vi "Find Invalid Group Settings.vi"(8 "error in (no error)":errorcluster, 11 "dsf refnum":T1) -> (0 "error out":errorcluster, 1 "Invalid Settings":string[](array[string]), 3 "dsf refnum out":T1)   [LabVIEW 2017, in "DSF Configuration.lvlib"]
uses:
  DSF Configuration.lvlib
  Controls/DSF Config Data RefNum.ctl
  Read All Item IDs/Read All Group IDs.vi
  Read Item Settings ID/Read Group Settings ID.vi
  Read All Item IDs/Read All Settings IDs.vi
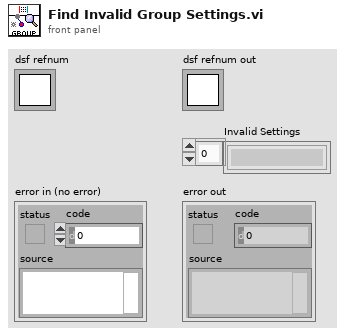
[diagram p1: front panel]
types:
  T1 = typedef "DSF Configuration.lvlib/DSF Config Data RefNum.ctl" = refnum<k1>
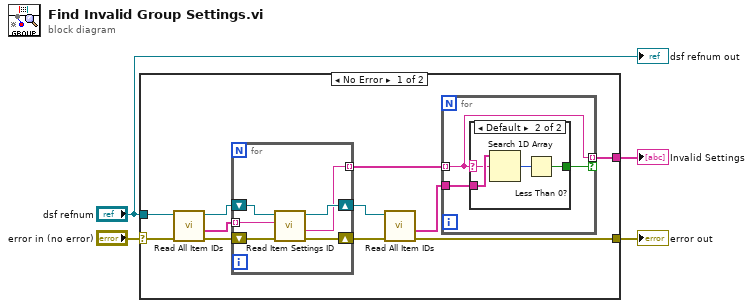
[diagram p0: block diagram]
diagram:
  n1 = case shown="No Error" "error in (no error)" {
    selector: "error in (no error)" -> [w15 w29]
    tunnel: "dsf refnum" -> [w14 _]
    tunnel: [w11 w29] -> w2
    tunnel: [w12 _] -> w1
    frame No Error {
      n2 = call-poly "Read All Item IDs.vi"("error in (no error)"=w15, "dsf refnum"=w14) -> ("error out"=w8:errorcluster, "Group IDs"=w6:string[], "dsf refnum out"=w10:T1)  [unwired: 7 in]
      n3 = for {
        shift-right: [w20] -> w9
        shift-left: w10 -> [w21]
        shift-right: [w18] -> w7
        shift-left: w8 -> [w19]
        tunnel: w6 -> [w17] mode=indexing
        tunnel: [w16] -> w5 mode=indexing
        n4 = call-poly "Read Item Settings ID.vi"("error in (no error)"=w19, "Group ID"=w17, "dsf refnum"=w21) -> ("error out"=w18:errorcluster, "Settings ID"=w16:string, "dsf refnum out"=w20:T1)  [unwired: 5 in, 1 out]
      }
      n5 = call-poly "Read All Item IDs.vi"("error in (no error)"=w7, "dsf refnum"=w9) -> ("error out"=w11:errorcluster, "Setting IDs"=w13:string[])  [unwired: 7 in, 1 out]
      n6 = for {
        tunnel: w5 -> [w23] mode=indexing
        tunnel: w13 -> [w24]
        tunnel: [w23] -> w12 mode=indexing if=w22
        n7 = case shown="Default" w23 {
          selector: w23 -> [_ w26]
          tunnel: w24 -> [_ w28]
          tunnel: [_ w25] -> w22
          frame "" {
          }
          frame Default {
            n8 = Search 1D Array(1D array=w28, element=w26) -> (index of element=w27:i32)  [unwired: 1 in]
            n9 = Less Than 0?(x=w27) -> (x < 0?=w25:bool)
          }
        }
      }
    }
    frame Error {
    }
  }
  "error out" <- w2
  "Invalid Settings" <- w1
  "dsf refnum out" <- "dsf refnum"
